vi "Main_menu.vi"() -> ()   [LabVIEW 2022 SP3]
doc: "The main menu function acts as the focal point for navigating and utilizing the diverse range of features and capabilities within our application. When users initiate the application, they encounter a user-friendly menu interface, offering a variety of options that cater to their specific requirements.\n Key functionalities include:\n Initiating window plots for data visualization\n Establishing communication with microcontrollers\n Implementing robust error handling mechanisms"
uses:
  <vilib>/event_ctls.llb/lveventtype.ctl
  <vilib>/Utility/file.llb/Write Delimited Spreadsheet (DBL).vi
panel:
  out "Cycle\ntime (ms)":u32
  in  "Clear error":bool
  out "Error":bool
  out "Close":bool
  in  "?":T1(tab)
  in  "New_plot_window":bool
  in  "List of active windows":i32(listbox)
  in  "Close all plots":bool
  in  "CSV Path for Signals":path
  in  "One time":i32
  out "Trace total samples":i32
  in  "Start record":bool
  in  "Continuous":i32
  in  "Global Mode":enum32{"Item 0", "Item 1"}(radio)
  in  "Samples per signal":u32
  in  "Trace names":string(combo)
  out "Total number signals":i32
  in  "Save CSV":bool
  in  "Stop":bool
  out "Run_record":bool
  in  "CTRL enable":bool
  in  "Save CTRL parameters":bool
  out "Total\ncontrols":i32
  in  "# Control":string(combo)
  in  "CS enable":bool
  out "CS status":i32
  in  "CS_IF_Params":T2 {"CS_Duty" min=0 max=1}
  out "Connected":bool
  out "Saved":bool
  in  "Save configuration":bool
  in  "Port":i32
  in  "Hostname":string
  in  "Timeout ms":i32
  in  "Send message":bool
  in  "Index window":i32
  in  "msj":string
  out "error out":errorcluster
  # "Refresh time (ms)"
  # "ctrl_if:0\nctrl: 2\nset parm: 2"
  # "In this section the user can send a message or data to a defined active window plot. \nJust to develop."
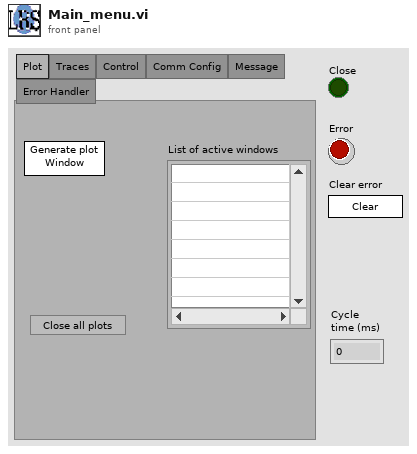
[diagram p1: front panel]
types:
  T1 = enum32{"Plot", "Traces", "Control", "Comm Config", "Message", "Error Handler"}
  T2 = cluster{"SET_PARAMETERS":i32, "CTLR":i32, "CS_Duty":sgl, "CTRL_IF_SET":i32}
  T3 = cluster{"Port":i32, "hostname":string, "status":bool, "timeout ms":i32, "TRACES_NAMES":string[], "Refresh time ms":i32, "Mode":enum32{"Item 0", "Item 1"}, "Start":bool, "DATA":sgl[][], "SIGNALS_NAMES":string[], "NB_SIGNALS":i32, "NB_TRACES":i32, "ID_TRACE":i32, "Mark":bool, "Counter":i32, "CTRLs_NAMES":string[], "NB_Ctrls":i32, "CS enable?":bool, "CS ID":i32}
  T4 = enum8{"Enabled", "Disabled", "Disabled and Grayed Out"}
  T5 = typedef "lveventtype.ctl" = enum32{"Null", "Timeout", "Annotation Menu Selection", "Annotation Menu Selection?", "App Instance Close", "App Instance Close?", "Autoscale Range Change", "Bookmark Info Change", "Cell Edit", "Cell Edit?", "Cursor Grab", "Cursor Grab?", "Cursor Menu Selection", "Cursor Menu Selection?", "Cursor Move", "Cursor Release", "Data Change", "Direction Change", "Display State Change", "Drag Ended", "Drag Enter", "Drag Leave", "Drag Over", "Drag Source Update", "Drag Starting", "Drag Starting?", "Drop", "Exec State Change", "Key Down", "Key Down?", "Key Repeat", "Key Repeat?", "Key Up", "Listbox Double Click", "Menu Activation?", "Menu Selection (App)", "Menu Selection? (App)", "Menu Selection (User)", "Mouse Down", "Mouse Down?", "Mouse Enter", "Mouse Leave", "Mouse Move", "Mouse Up", "Mouse Wheel", "NI Security User Change (App)", "Pane Size", "Panel Close", "Panel Close?", "Panel Resize", "Plot Attribute Change", "Scale Range Change", "Shortcut Menu Activation?", "Shortcut Menu Selection (App)", "Shortcut Menu Selection? (App)", "Shortcut Menu Selection (User)", "Tree Double Click", "Tree Drag", "Tree Drag?", "Tree Drop", "Tree Drop?", "Tree Item Close", "Tree Item Close?", "Tree Item Open", "Tree Item Open?", "User Event", "Value Change"}
  T6 = enum16{"open", "replace", "create", "open or create", "replace or create", "replace or create with confirmation"}
  T7 = enum32{"Invalid", "Standard", "Closed", "Hidden", "Minimized", "Maximized"}
  T8 = enum32{"invalid app kind", "Development System", "Run Time System", "Student Edition", "Embedded LabVIEW", "Evaluation", "Custom"}
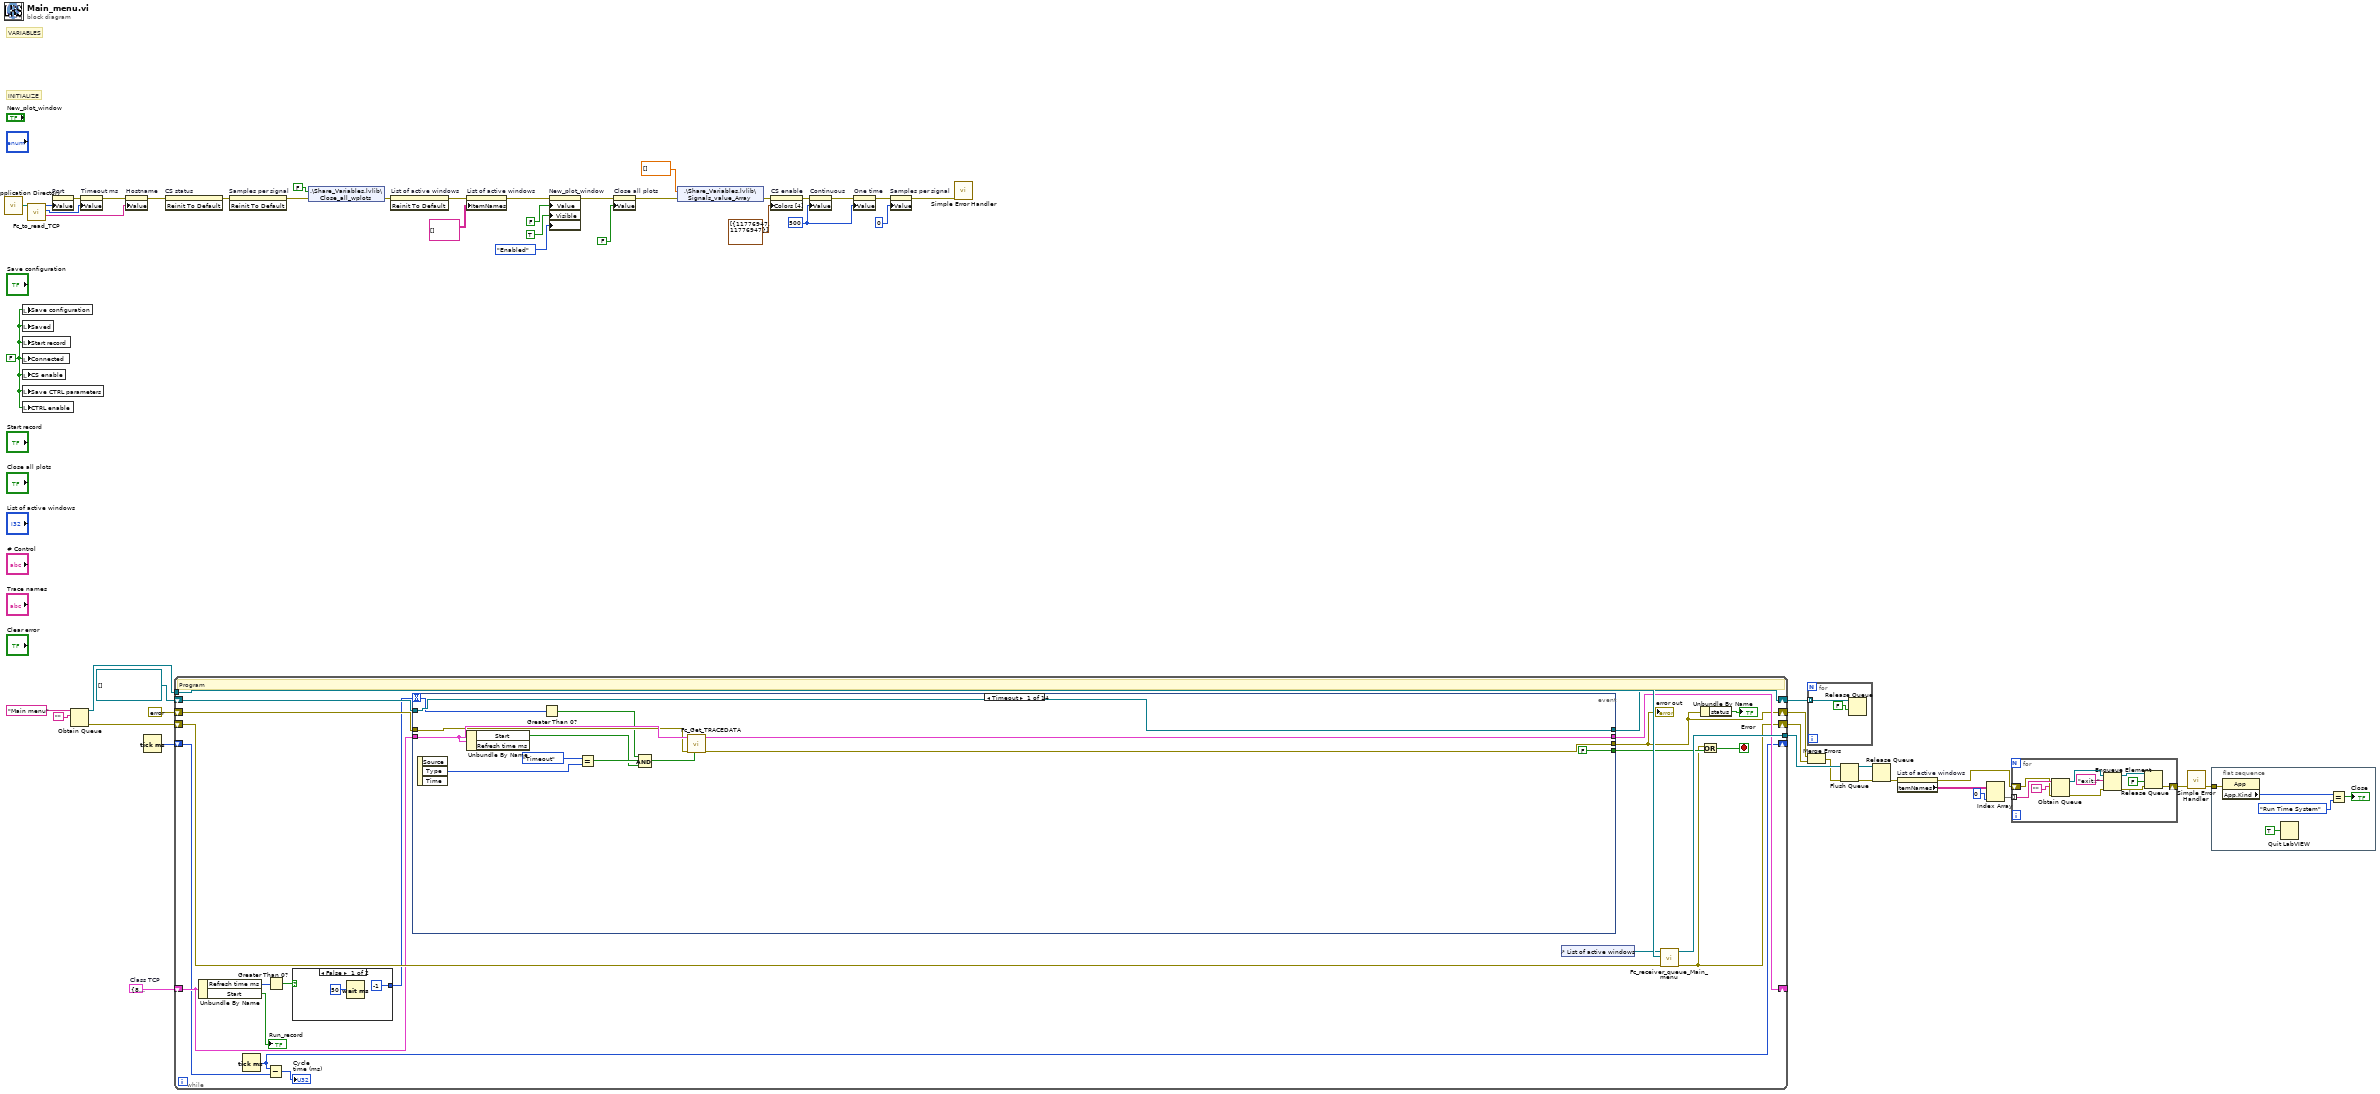
[diagram p0: block diagram]
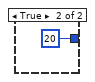
[diagram p2: hidden frame]
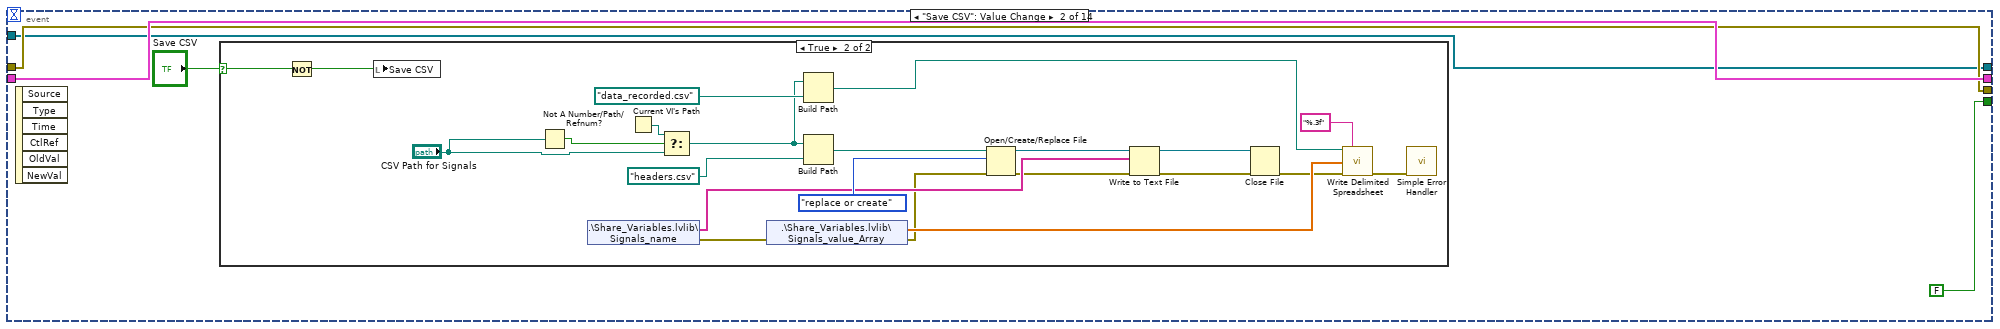
[diagram p3: hidden frame]
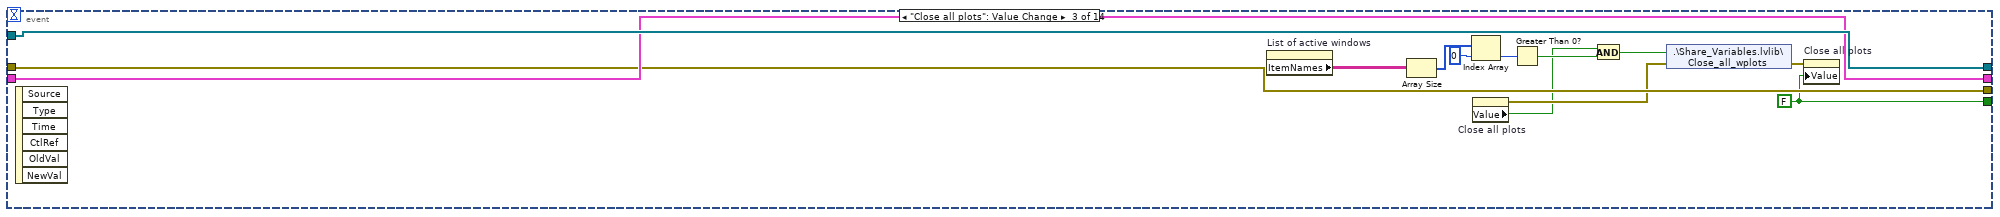
[diagram p5: hidden frame]
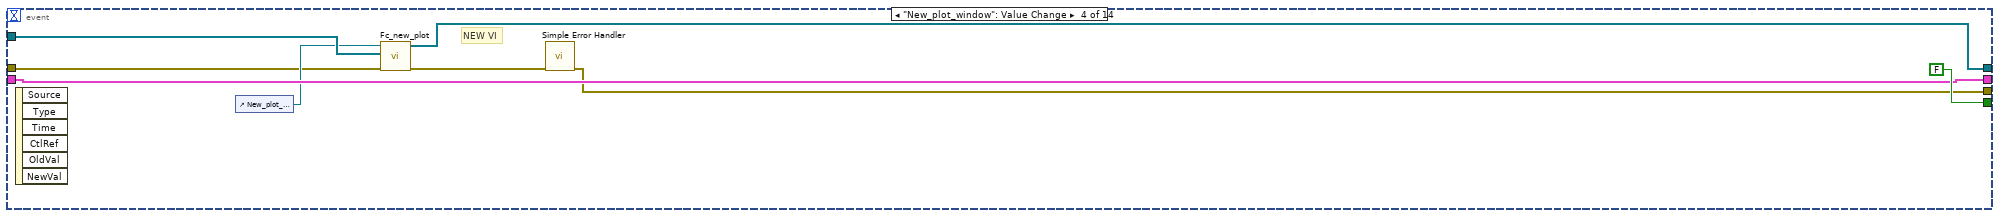
[diagram p6: hidden frame]
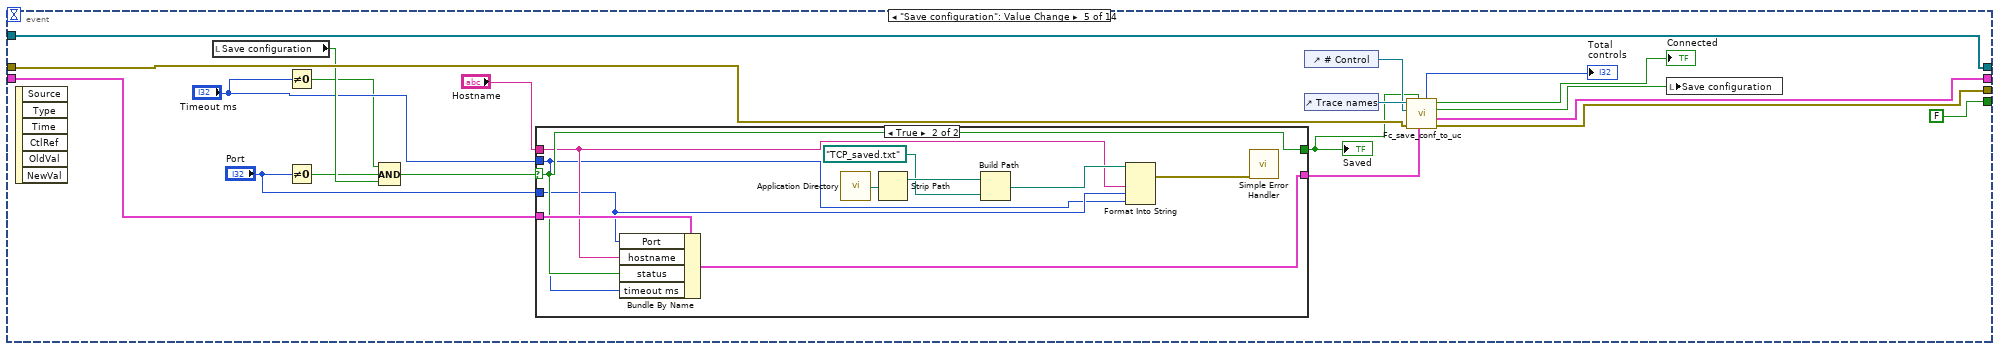
[diagram p7: hidden frame]
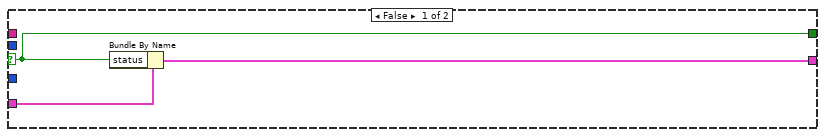
[diagram p8: hidden frame]
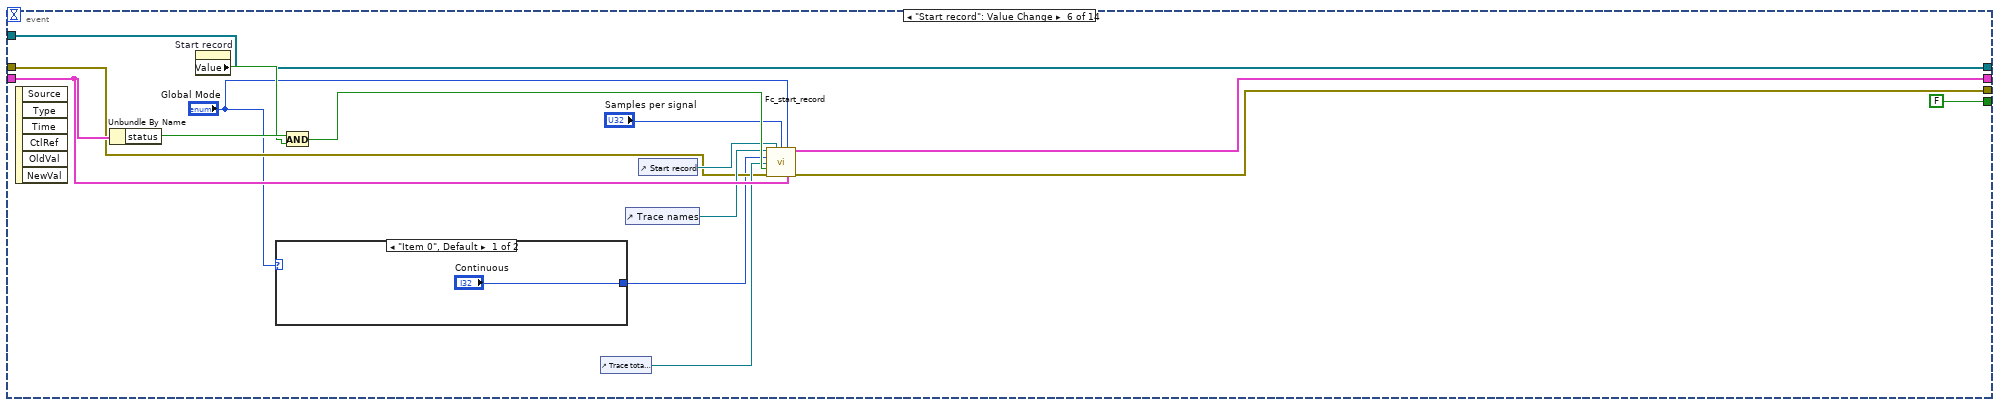
[diagram p9: hidden frame]
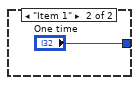
[diagram p10: hidden frame]
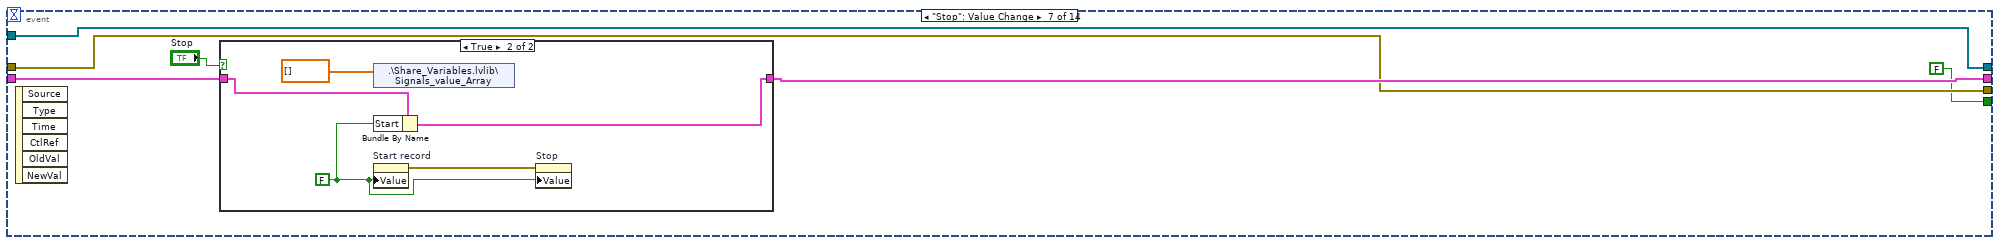
[diagram p11: hidden frame]
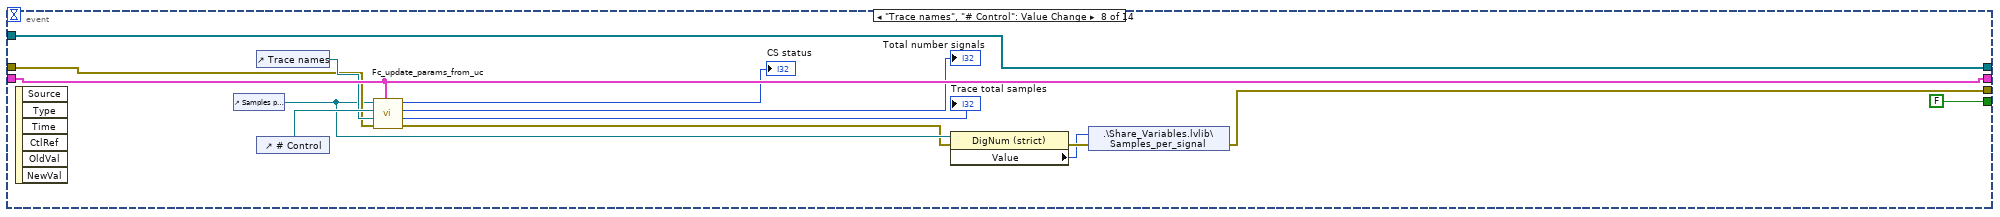
[diagram p13: hidden frame]
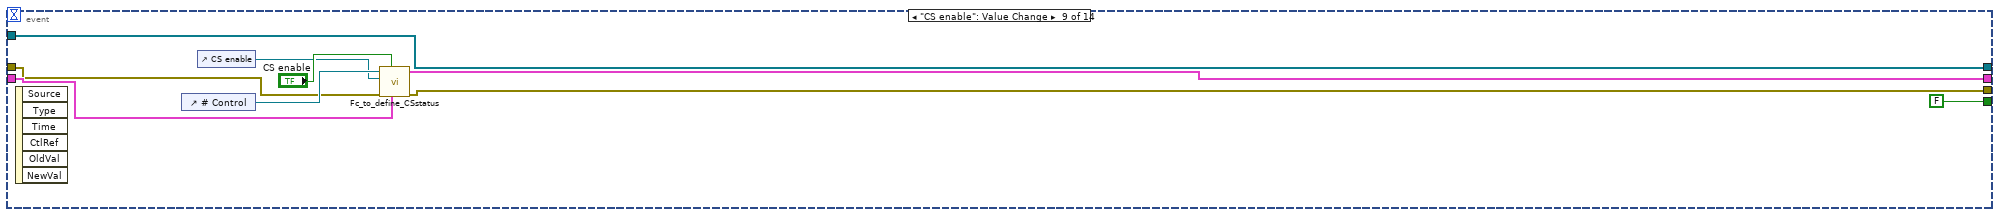
[diagram p14: hidden frame]
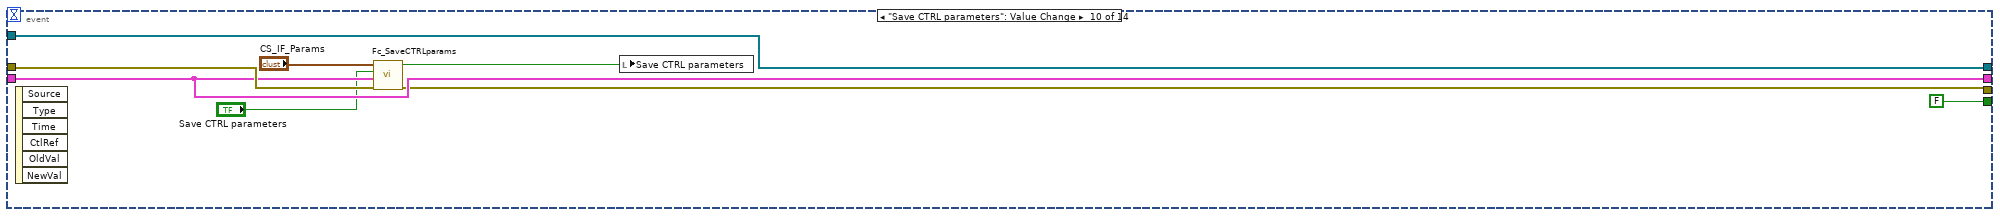
[diagram p15: hidden frame]
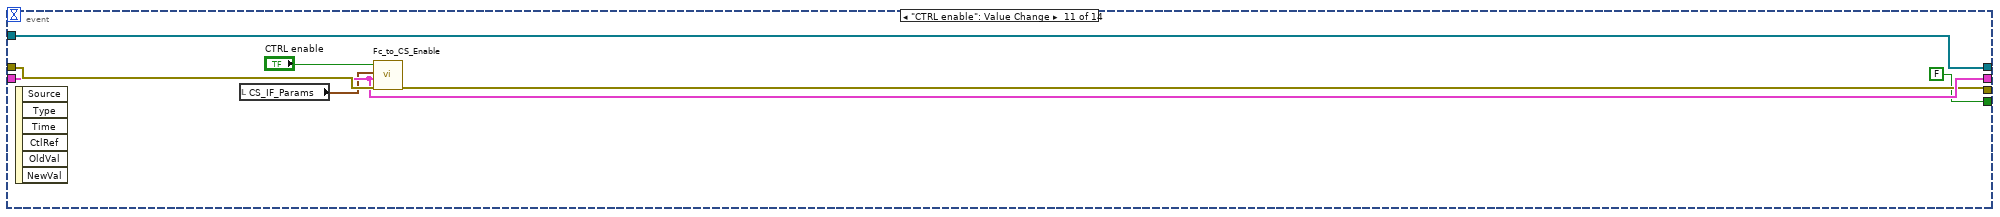
[diagram p16: hidden frame]
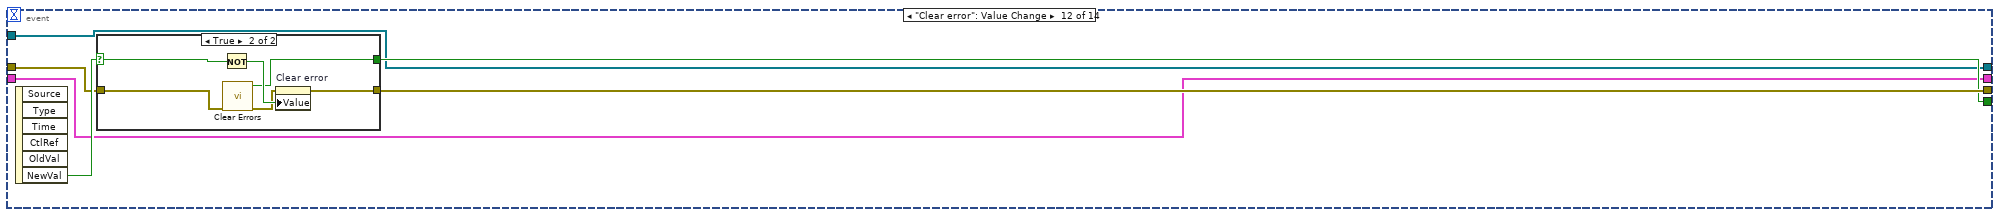
[diagram p17: hidden frame]
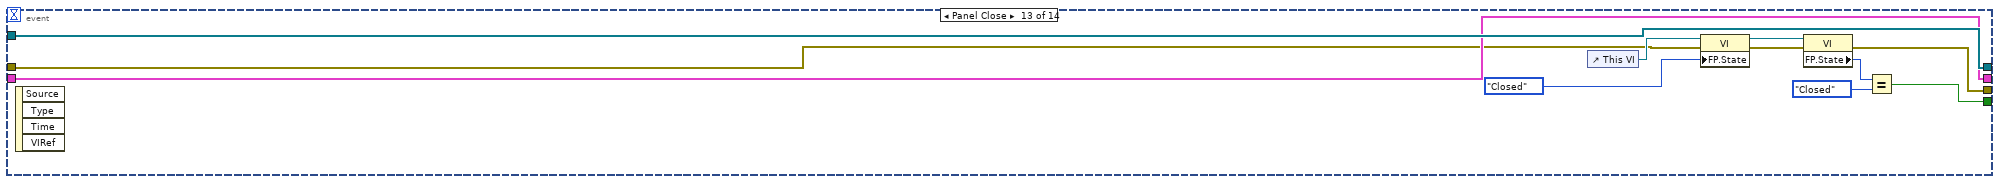
[diagram p19: hidden frame]
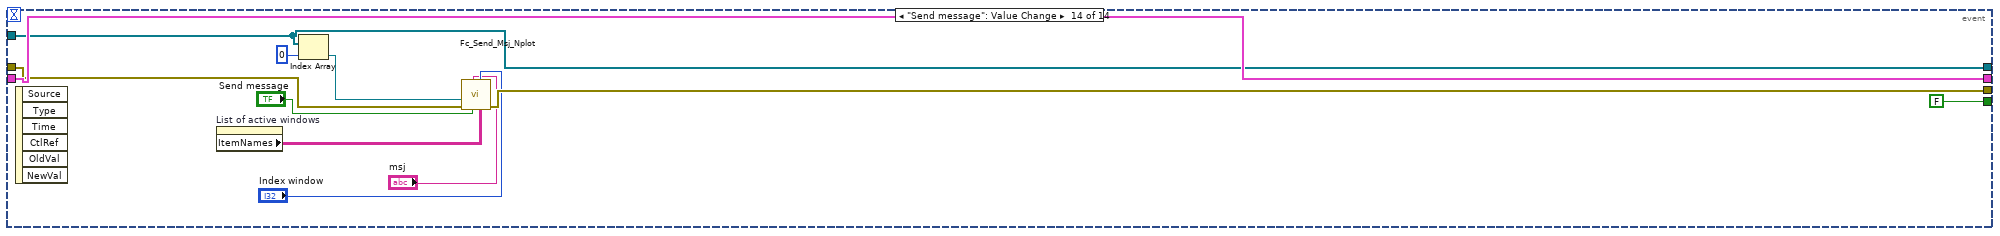
[diagram p20: hidden frame]
diagram:
  w14 = 500 ("Refresh \ntime (ms)")
  w34 = T3 {"Port"=8085, "hostname"="", "status"=FALSE, "timeout ms"=1000, "TRACES_NAMES"=[], "Refresh time ms"=-1, "Mode"=enum."Item 0", "Start"=FALSE, "DATA"=[], "SIGNALS_NAMES"=[], "NB_SIGNALS"=0, "NB_TRACES"=0, "ID_TRACE"=0, "Mark"=FALSE, "Counter"=0, "CTRLs_NAMES"=[], "NB_Ctrls"=0, "CS enable?"=FALSE, "CS ID"=0}  # Class TCP
  w23 = FALSE ("Save conf")
  # "INITIALIZE"
  # "VARIABLES"
  n1 = call <vilib>:"Application Directory.vi"() -> ("Application Directory"=w7:path)
  n2 = local write "Save configuration"(w23) -> ()
  n3 = local write "Saved"(w23) -> ()
  n4 = local write "Start record"(w23) -> ()
  n5 = local write "Connected"(w23) -> ()
  n6 = local write "CS enable"(w23) -> ()
  n7 = local write "Save CTRL parameters"(w23) -> ()
  n8 = local write "CTRL enable"(w23) -> ()
  n9 = call "Fc_to_read_TCP.vi"("path_mainmenu"=w7) -> ("Hhostname"=w10:string, "Timeout ms"=w8:i32, "Port"=w9:i32)  [unwired: 8 in]
  n10 = property on="Port" class="DigNum (strict)"("Value"=w9) -> (error out=w33:errorcluster)  [unwired: 2 in, 1 out]
  n11 = Obtain Queue(name (unnamed)="Main menu", element data type="") -> (queue out=w45:refnum<queue>, error out=w44:errorcluster)  [unwired: 3 in, 1 out]
  n12 = property on="Timeout ms" class="DigNum (strict)"(error in=w33, "Value"=w8) -> (error out=w29:errorcluster)  [unwired: 1 in, 1 out]
  n13 = property on="Hostname" class="Str"(error in=w29, "Value"=w10) -> (error out=w19:errorcluster)  [unwired: 1 in, 1 out]
  n14 = Tick Count (ms)() -> (millisecond timer value=w6:u32)
  n15 = invoke on="CS status" class="DigNum (strict)" method="Reinit To Default"(error in=w19) -> (error out=w28:errorcluster)  [unwired: 2 in, 2 out]
  n16 = while {
    shift-right: [w67] -> w49
    shift-left: refnum<queue>[] [] -> [w73]
    tunnel: w45 -> [w72]
    tunnel: [w71] -> w37
    shift-right: [w61] -> w5
    shift-left: w44 -> [w70]
    shift-right: [w69] -> _
    shift-left: w34 -> [w68]
    shift-right: [w64] -> w1
    shift-left: errorcluster {"status"=FALSE, "code"=0, "source"=""} ("error out") -> [w65]
    shift-right: [w54] -> _
    shift-left: w6 -> [w55]
    stop <- w62 stop-if-true
    # "Program"
    n17 = Unbundle By Name(w68) -> ("Refresh time ms"=w58:i32, "Start"=→"Run_record":bool)
    n18 = Tick Count (ms)() -> (millisecond timer value=w54:u32)
    n19 = Subtract(x=w54, y=w55) -> (x-y=→"Cycle\ntime (ms)":u32)
    n20 = Greater Than 0?(x=w58) -> (x > 0?=w59:bool)
    n21 = case shown="False" w59 {
      tunnel: [-1 20] -> w57
      frame False {
        n22 = Wait (ms)(milliseconds to wait=u32 50) -> ()  [unwired: 1 out]
      }
      frame True {
      }
    }
    n23 = event shown="[0] Timeout" {
      selector: _ -> [_ _ _ _ _ _ _ _ _ _ _ _ _ _]
      dyn-events: _ -> [_ _ _ _ _ _ _ _ _ _ _ _ _ _]
      timeout: w57 -> [w81 _ _ _ _ _ _ _ _ _ _ _ _ _]
      tunnel: [FALSE ("f") FALSE ("specific error cleared?") w120 FALSE ("f") FALSE ("f") FALSE ("f") FALSE ("specific error cleared?") FALSE ("f") FALSE ("specific error cleared?") FALSE ("specific error cleared?") FALSE ("specific error cleared?") w241 w261 FALSE ("specific error cleared?")] -> w63
      tunnel: [w89 w91 w129 w137 w143 w173 w190 w206 w216 w225 w233 w239 w260 w269] -> w67
      tunnel: w73 -> [w89 w91 w129 w136 w143 w173 w190 w206 w216 w225 w233 w239 w260 w269]
      tunnel: [w85 w93 w124 w134 w152 w183 w192 w213 w223 w230 w237 w240 w256 w274] -> w69
      tunnel: w68 -> [w86 w93 w124 w134 w157 w184 w193 w213 w222 w230 w237 w240 w256 w274]
      tunnel: w65 -> [w83 w92 w123 w132 w155 w177 w191 w207 w219 w231 w238 w243 w254 w272]
      tunnel: [w82 w92 w123 w130 w144 w176 w191 w201 w217 w226 w234 w242 w253 w271] -> w64
      event Timeout {
        n24 = event-data() -> ("Type"=w87:T5)  [unwired: 1 in, 2 out]
        n25 = Unbundle By Name(w86) -> ("Start"=w78:bool)  [unwired: 1 out]
        n26 = Greater Than 0?(x=w81) -> (x > 0?=w80:bool)
        n27 = Equal?(x=lveventtype."Timeout" ("Type"), y=w87) -> (x = y?=w79:bool)
        n28 = Compound Arithmetic op=AND(w80, w79, w78) -> (w77:bool)
        n29 = call "Fc_Get_TRACEDATA.vi"("Start+timeout?"=w77, "error in (no error)"=w83, "Class TCP in"=w86) -> ("error out"=w82:errorcluster, "Class TCP out"=w85:T3)  [unwired: 7 in]
      }
      event "Save CSV": Value Change {
        n30 = event-data() -> ()  [unwired: 1 in, 6 out]
        n31 = case shown="True" "Save CSV" {
          selector: "Save CSV" -> [_ w98]
          frame False {
          }
          frame True {
            n32 = Not(x=w98) -> (.not. x?=w97:bool)
            n33 = local write "Save CSV"(w97) -> ()
            n34 = Not A Number/Path/Refnum?(number/path/refnum="CSV Path for Signals") -> (NaN/Path/Refnum?=w102:bool)
            n35 = shared-variable ".\\Share_Variables.lvlib\\Signals_name"() -> (w107:string[], error out=w96:errorcluster)  [unwired: 1 in]
            n36 = Current VI's Path() -> (path=w101:path)
            n37 = Select(t=w101, s=w102, f="CSV Path for Signals") -> (s? t:f=w99:path)
            n38 = shared-variable ".\\Share_Variables.lvlib\\Signals_value_Array"(error in=w96) -> (w113:dbl[], error out=w95:errorcluster)
            n39 = Build Path(base path=w99, name or relative path=path "data_recorded.csv") -> (appended path=w112:path)
            n40 = Build Path(base path=w99, name or relative path=path "headers.csv") -> (appended path=w110:path)
            n41 = Open/Create/Replace File(file path (use dialog)=w110, error in=w95, operation (0:open)=T6."replace or create") -> (refnum out=w108:refnum<file>, error out=w105:errorcluster)  [unwired: 3 in, 1 out]
            n42 = Write to Text File(file (use dialog)=w108, text=w107, error in=w105) -> (refnum out=w106:refnum<file>, error out=w104:errorcluster)  [unwired: 1 in, 1 out]
            n43 = Close File(refnum=w106, error in=w104) -> (error out=w103:errorcluster)  [unwired: 1 out]
            n44 = call-poly <vilib>:"Write Delimited Spreadsheet.vi"("file path (dialog if empty)"=w112, "format (%.3f)"="%.3f", "1D data"=w113, "error in (no error)"=w103) -> ("error out"=w114:errorcluster)  [unwired: 10 in, 1 out]
            n45 = call <vilib>:"Simple Error Handler.vi"("error in (no error)"=w114) -> ()  [unwired: 4 in, 5 out]
          }
        }
      }
      event "Close all plots": Value Change {
        w120 = FALSE ("f")
        n46 = event-data() -> ()  [unwired: 1 in, 6 out]
        n47 = property on="List of active windows" class="MCListbox (strict)"() -> ("ItemNames"=w125:string[][])  [unwired: 2 in, 2 out]
        n48 = Array Size(array=w125) -> (size(s)=w128:i32[])
        n49 = Index Array(array=w128, index=0) -> (element=w126:i32)
        n50 = property on="Close all plots" class="Bool (strict)"() -> (error out=w118:errorcluster, "Value"=w117:bool)  [unwired: 2 in, 1 out]
        n51 = Greater Than 0?(x=w126) -> (x > 0?=w119:bool)
        n52 = And(x=w117, y=w119) -> (x .and. y?=w122:bool)
        n53 = shared-variable ".\\Share_Variables.lvlib\\Close_all_wplots"(w122, error in=w118) -> (error out=w121:errorcluster)
        n54 = property on="Close all plots" class="Bool (strict)"(error in=w121, "Value"=w120) -> ()  [unwired: 1 in, 2 out]
      }
      event "New_plot_window": Value Change {
        # "NEW VI"
        n55 = event-data() -> ()  [unwired: 1 in, 6 out]
        n56 = control-ref of="New_plot_window"() -> (w133:refnum<vi>)
        n57 = call "Fc_new_plot.vi"("error in (no error)"=w132, "Array in"=w136, "Boolean in"=w133) -> ("error out"=w131:errorcluster, "Array out"=w137:refnum<queue>[])  [unwired: 7 in]
        n58 = call <vilib>:"Simple Error Handler.vi"("error in (no error)"=w131) -> ("error out"=w130:errorcluster)  [unwired: 4 in, 4 out]
      }
      event "Save configuration": Value Change {
        n59 = event-data() -> ()  [unwired: 1 in, 6 out]
        n60 = local read "Save configuration"() -> (w146:bool)
        n61 = Not Equal To 0?(x="Timeout ms") -> (x != 0?=w140:bool)
        n62 = Not Equal To 0?(x="Port") -> (x != 0?=w139:bool)
        n63 = Compound Arithmetic op=AND(w140, w139, w146) -> (w145:bool)
        n64 = case shown="True" w145 {
          selector: w145 -> [w158 w169]
          tunnel: [w158 w169] -> w142
          tunnel: "Port" -> [_ w164]
          tunnel: "Hostname" -> [_ w165]
          tunnel: [w160 w170] -> w153
          tunnel: w157 -> [w159 w171]
          tunnel: "Timeout ms" -> [_ w163]
          frame False {
            n65 = Bundle By Name(cluster=w159, "status"=w158) -> (w160:T3)
          }
          frame True {
            n66 = Bundle By Name(cluster=w171, "Port"=w164, "hostname"=w165, "status"=w169, "timeout ms"=w163) -> (w170:T3)
            n67 = call <vilib>:"Application Directory.vi"() -> ("Application Directory"=w161:path)
            n68 = Strip Path(path=w161) -> (stripped path=w168:path)  [unwired: 1 out]
            n69 = Build Path(base path=w168, name or relative path=path "TCP_saved.txt" ("default name")) -> (appended path=w166:path)
            n70 = Format Into String(initial string=w166, w165, w164, w163) -> (error out=w162:errorcluster)  [unwired: 2 in, 1 out]
            n71 = call <vilib>:"Simple Error Handler.vi"("error in (no error)"=w162) -> ()  [unwired: 4 in, 5 out]
          }
        }
        "Saved" <- w142
        n72 = control-ref of="# Control"() -> (w147:refnum<vi>)
        n73 = control-ref of="Trace names"() -> (w148:refnum<vi>)
        n74 = call "Fc_save_conf_to_uc.vi"("Class TCP in"=w153, "Saved configuration?"=w142, "error in (no error)"=w155, "# Control Refnum in"=w147, "Trace names Refnum in"=w148) -> ("error out"=w144:errorcluster, "Class TCP out"=w152:T3, "Save conf?"=w154:bool, "Connected?"=→"Connected":bool, "NB_CSs"=→"Total\ncontrols":i32)  [unwired: 2 in]
        n75 = local write "Save configuration"(w154) -> ()
      }
      event "Start record": Value Change {
        n76 = event-data() -> ()  [unwired: 1 in, 6 out]
        n77 = Unbundle By Name(w184) -> ("status"=w186:bool)
        n78 = property on="Start record" class="Bool (strict)"() -> ("Value"=w181:bool)  [unwired: 2 in, 2 out]
        n79 = case shown="\"Item 0\", Default" "Global Mode" {
          tunnel: ["Continuous" "One time"] -> w174
          frame "Item 0", Default {
          }
          frame "Item 1" {
          }
        }
        n80 = And(x=w186, y=w181) -> (x .and. y?=w185:bool)
        n81 = control-ref of="Trace total samples"() -> (w178:refnum<vi>)
        n82 = control-ref of="Trace names"() -> (w180:refnum<vi>)
        n83 = control-ref of="Start record"() -> (w179:refnum<vi>)
        n84 = call "Fc_start_record.vi"("Trace names"=w180, "Start record?"=w179, "Samples X Signal"="Samples per signal", "Global Mode"="Global Mode", "Refresh \ntime (ms)"=w174, "total samples?"=w178, "status+start record"=w185, "error in (no error)"=w177, "Class TCP in"=w184) -> ("Class TCP out"=w183:T3, "error out"=w176:errorcluster)  [unwired: 5 in]
      }
      event "Stop": Value Change {
        n85 = event-data() -> ()  [unwired: 1 in, 6 out]
        n86 = case shown="True" "Stop" {
          tunnel: w193 -> [w195 w200]
          tunnel: [w195 w196] -> w192
          frame False {
          }
          frame True {
            w197 = FALSE ("Start")
            n87 = shared-variable ".\\Share_Variables.lvlib\\Signals_value_Array"(dbl[] [] ("Signals_value_Array")) -> ()  [unwired: 1 in, 1 out]
            n88 = Bundle By Name(cluster=w200, "Start"=w197) -> (w196:T3)
            n89 = property on="Start record" class="Bool (strict)"("Value"=w197) -> (error out=w198:errorcluster)  [unwired: 2 in, 1 out]
            n90 = property on="Stop" class="Bool (strict)"(error in=w198, "Value"=w197) -> ()  [unwired: 1 in, 2 out]
          }
        }
      }
      event "Trace names", "# Control": Value Change {
        n91 = event-data() -> ()  [unwired: 1 in, 6 out]
        n92 = control-ref of="Samples per signal"() -> (w205:refnum<vi>)
        n93 = control-ref of="Trace names"() -> (w208:refnum<vi>)
        n94 = control-ref of="# Control"() -> (w209:refnum<vi>)
        n95 = call "Fc_update_params_from_uc.vi"("Class TCP"=w213, "error in (no error)"=w207, "Trace names"=w208, "# Control"=w209, "SamplesPerSignal?"=w205) -> ("error out"=w202:errorcluster, "TRACE_SIZE"=→"Trace total samples":i32, "NB_TRACED_SIGNALS"=→"Total number signals":i32, "CS STATUS"=→"CS status":i32)  [unwired: 3 in]
        n96 = property class="DigNum (strict)"(reference=w205, error in=w202) -> (error out=w204:errorcluster, "Value"=w203:u32)  [unwired: 1 out]
        n97 = shared-variable ".\\Share_Variables.lvlib\\Samples_per_signal"(w203, error in=w204) -> (error out=w201:errorcluster)
      }
      event "CS enable": Value Change {
        n98 = event-data() -> ()  [unwired: 1 in, 6 out]
        n99 = control-ref of="# Control"() -> (w220:refnum<vi>)
        n100 = control-ref of="CS enable"() -> (w218:refnum<vi>)
        n101 = call "Fc_to_define_CSstatus.vi"("Class TCP in"=w222, 7:"CS enable"="CS enable", "error in (no error)"=w219, 10:"CS enable"=w218, "# Control?"=w220) -> ("error out"=w217:errorcluster, "Class TCP out"=w223:T3)  [unwired: 5 in]
      }
      event "Save CTRL parameters": Value Change {
        n102 = event-data() -> ()  [unwired: 1 in, 6 out]
        n103 = call "Fc_SaveCTRLparams.vi"("error in (no error)"=w231, "Class TCP"=w230, "Save CTRL params"="Save CTRL parameters", "CS_IF_Params"="CS_IF_Params") -> ("error out"=w226:errorcluster, "Saved CTRL params ?"=w227:bool)  [unwired: 6 in]
        n104 = local write "Save CTRL parameters"(w227) -> ()
      }
      event "CTRL enable": Value Change {
        n105 = event-data() -> ()  [unwired: 1 in, 6 out]
        n106 = local read "CS_IF_Params"() -> (w235:T2)
        n107 = call "Fc_to_CS_Enable.vi"("error in (no error)"=w238, "Class TCP"=w237, "CS_IF_Params"=w235, "CTRL enable"="CTRL enable") -> ("error out"=w234:errorcluster)  [unwired: 7 in]
      }
      event "Clear error": Value Change {
        n108 = event-data() -> ("NewVal"=w244:bool)  [unwired: 1 in, 5 out]
        n109 = case shown="True" w244 {
          selector: w244 -> [w245 w252]
          tunnel: w243 -> [w246 w249]
          tunnel: [w246 w247] -> w242
          tunnel: [w245 w250] -> w241
          frame False {
          }
          frame True {
            n110 = Not(x=w252) -> (.not. x?=w251:bool)
            n111 = call <vilib>:"Clear Errors.vi"("error in (no error)"=w249) -> ("error out"=w248:errorcluster, "specific error cleared?"=w250:bool)  [unwired: 5 in]
            n112 = property on="Clear error" class="Bool (strict)"(error in=w248, "Value"=w251) -> (error out=w247:errorcluster)  [unwired: 1 in, 1 out]
          }
        }
      }
      event Panel Close {
        n113 = event-data() -> ()  [unwired: 1 in, 4 out]
        n114 = control-ref of="This VI"() -> (w259:refnum<vi>)
        n115 = property class="VI"(reference=w259, error in=w254, "FP.State"=T7."Closed" ("Front Panel Window:State")) -> (reference out=w258:refnum<vi>, error out=w255:errorcluster)
        n116 = property class="VI"(reference=w258, error in=w255) -> (error out=w253:errorcluster, "FP.State"=w263:T7)  [unwired: 1 out]
        n117 = Equal?(x=w263, y=T7."Closed") -> (x = y?=w261:bool)
      }
      event "Send message": Value Change {
        n118 = event-data() -> ()  [unwired: 1 in, 6 out]
        n119 = property on="List of active windows" class="MCListbox (strict)"() -> ("ItemNames"=w266:string[][])  [unwired: 2 in, 2 out]
        n120 = Index Array(array=w269, index=0) -> (element=w268:refnum<queue>)
        n121 = call "Fc_Send_Msj_Nplot.vi"("ItemNames"=w266, "Process in"="Index window", "Send message"="Send message", "msj"="msj", "error in (no error)"=w272, "queue in"=w268) -> ("error out"=w271:errorcluster)  [unwired: 5 in]
      }
    }
    "error out" <- w64
    n122 = control-ref of="List of active windows"() -> (w66:refnum<vi>)
    n123 = call "Fc_receiver_queue_Main_menu.vi"("error in (no error)"=w70, "Queue in"=w72, "MulticolumnListbox in"=w66) -> ("error out"=w61:errorcluster, "Queue out"=w71:refnum<queue>)  [unwired: 7 in]
    n124 = Unbundle By Name(w64) -> ("status"=→"Error":bool)
    n125 = Or(x=w61, y=w63) -> (x .or. y?=w62:bool)
  }
  n126 = invoke on="Samples per signal" class="DigNum (strict)" method="Reinit To Default"(error in=w28) -> (error out=w27:errorcluster)  [unwired: 2 in, 2 out]
  n127 = shared-variable ".\\Share_Variables.lvlib\\Close_all_wplots"(FALSE ("Close_all_wplots"), error in=w27) -> (error out=w32:errorcluster)
  n128 = invoke on="List of active windows" class="MCListbox (strict)" method="Reinit To Default"(error in=w32) -> (error out=w35:errorcluster)  [unwired: 2 in, 2 out]
  n129 = property on="List of active windows" class="MCListbox (strict)"(error in=w35, "ItemNames"=string[][] [] ("Item Names")) -> (error out=w26:errorcluster)  [unwired: 1 in, 1 out]
  n130 = property on="New_plot_window" class="Bool (strict)"(error in=w26, "Value"=FALSE ("New plot"), "Visible"=TRUE, "DisabledEnum"=T4."Enabled" ("Disabled")) -> (error out=w25:errorcluster)  [unwired: 1 in, 1 out]
  n131 = property on="Close all plots" class="Bool (strict)"(error in=w25, "Value"=FALSE ("Cancel Button")) -> (error out=w18:errorcluster)  [unwired: 1 in, 1 out]
  n132 = shared-variable ".\\Share_Variables.lvlib\\Signals_value_Array"(dbl[] [] ("Signals_value_Array"), error in=w18) -> (error out=w22:errorcluster)
  n133 = property on="CS enable" class="Bool (strict)"(error in=w22, "Colors [4]"=cluster{u32, u32}[] [{11776947, 11776947}]) -> (error out=w20:errorcluster)  [unwired: 1 in, 1 out]
  n134 = property on="Continuous" class="DigNum (strict)"(error in=w20, "Value"=w14) -> (error out=w15:errorcluster)  [unwired: 1 in, 1 out]
  n135 = property on="One time" class="DigNum (strict)"(error in=w15, "Value"=w14) -> (error out=w13:errorcluster)  [unwired: 1 in, 1 out]
  n136 = property on="Samples per signal" class="DigNum (strict)"(error in=w13, "Value"=u32 0 ("Samples per signal")) -> (error out=w12:errorcluster)  [unwired: 1 in, 1 out]
  n137 = call <vilib>:"Simple Error Handler.vi"("error in (no error)"=w12) -> ()  [unwired: 4 in, 5 out]
  n138 = for {
    tunnel: w49 -> [w276] mode=indexing
    n139 = Release Queue(queue=w276, force destroy? (F)=FALSE) -> ()  [unwired: 1 in, 3 out]
  }
  n140 = Merge Errors(w1, w5) -> (w2:errorcluster)
  n141 = Flush Queue(queue=w37, error in (no error)=w2) -> (queue out=w3:refnum<queue>, error out=w4:errorcluster)  [unwired: 1 out]
  n142 = Release Queue(queue=w3, error in (no error)=w4) -> (error out=w16:errorcluster)  [unwired: 1 in, 2 out]
  n143 = property on="List of active windows" class="MCListbox (strict)"(error in=w16) -> (error out=w40:errorcluster, "ItemNames"=w43:string[][])  [unwired: 1 in, 1 out]
  n144 = Index Array(array=w43, index (col)=0 ("disabled index (col)")) -> (element=w41:string[])  [unwired: 1 in]
  n145 = for {
    tunnel: w41 -> [w286] mode=indexing
    shift-right: [w283] -> w39
    shift-left: w40 -> [w285]
    n146 = Obtain Queue(name (unnamed)=w286, element data type="", error in (no error)=w285) -> (queue out=w278:refnum<queue>, error out=w280:errorcluster)  [unwired: 2 in, 1 out]
    n147 = Enqueue Element(queue=w278, element="exit::", error in (no error)=w280) -> (queue out=w277:refnum<queue>, error out=w279:errorcluster)  [unwired: 1 in, 1 out]
    n148 = Release Queue(queue=w277, force destroy? (F)=FALSE, error in (no error)=w279) -> (error out=w283:errorcluster)  [unwired: 2 out]
  }
  n149 = call <vilib>:"Simple Error Handler.vi"("error in (no error)"=w39) -> ("error out"=w38:errorcluster)  [unwired: 4 in, 4 out]
  n150 = flat-sequence {
    tunnel: w38 -> [w287]
    frame #0 {
      n151 = property class="App"(error in=w287) -> ("App.Kind"=w291:T8)  [unwired: 1 in, 2 out]
      n152 = Quit LabVIEW(quit? (T)=TRUE) -> ()
      n153 = Equal?(x=w291, y=T8."Run Time System" ("Application:Kind")) -> (x = y?=→"Close":bool)
    }
  }
